vi "StopRxSession.vi"(8 "error in (no error)":errorcluster, 11 "NI-XNET in":refnum<class "NI-XNET.lvclass">) -> (0 "error out":errorcluster, 3 "NI-XNET out":refnum<class "NI-XNET.lvclass">)   [LabVIEW 2023, in "HardwareAbstractionLayer_LVOOP.lvlib" / "CAN HAL Lib.lvlib" / "NI-XNET.lvclass"]
uses:
  NI-XNET.lvclass
  NI-XNET.lvclass/NI-XNET.ctl
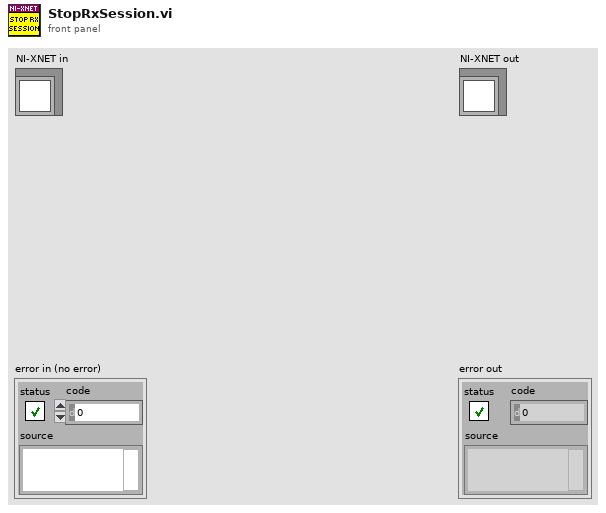
[diagram p1: front panel]
types:
  T1 = typedef "XNET Control Scope.ctl" = u32
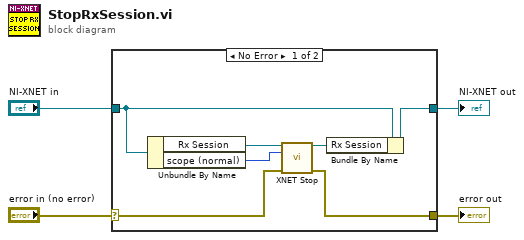
[diagram p0: block diagram]
diagram:
  n1 = case shown="No Error" "error in (no error)" {
    selector: "error in (no error)" -> [w10 w13]
    tunnel: [w8 w13] -> w2
    tunnel: [w7 w12] -> w1
    tunnel: "NI-XNET in" -> [w11 w12]
    frame No Error {
      n2 = Unbundle By Name(w11) -> ("Rx Session"=w9:refnum<k21>, "scope (normal)"=w5:T1)
      n3 = call <vilib>:"XNET Stop.vi"("session in"=w9, "scope (normal)"=w5, "error in (no error)"=w10) -> ("session out"=w6:refnum<k21>, "error out"=w8:errorcluster)  [unwired: 11 in]
      n4 = Bundle By Name(cluster=w11, "Rx Session"=w6) -> (w7:refnum<class "NI-XNET.lvclass">)
    }
    frame Error {
    }
  }
  "error out" <- w2
  "NI-XNET out" <- w1
